vi "FlattenFRF.vi"(9 "CrsrList":T1, 11 "Data in":cluster{"t0":dbl, "dt":dbl, "Y":cdb[]}) -> (1 "Data out":cluster{"t0":dbl, "dt":dbl, "Y":cdb[]})   [LabVIEW 2022 SP3]
uses:
  <vilib>/Utility/miscctls.llb/LVCursorListTypeDef.ctl
panel:
  out "FRF":cluster{"t0":dbl, "dt":dbl, "Y":dbl[]}[](graph)
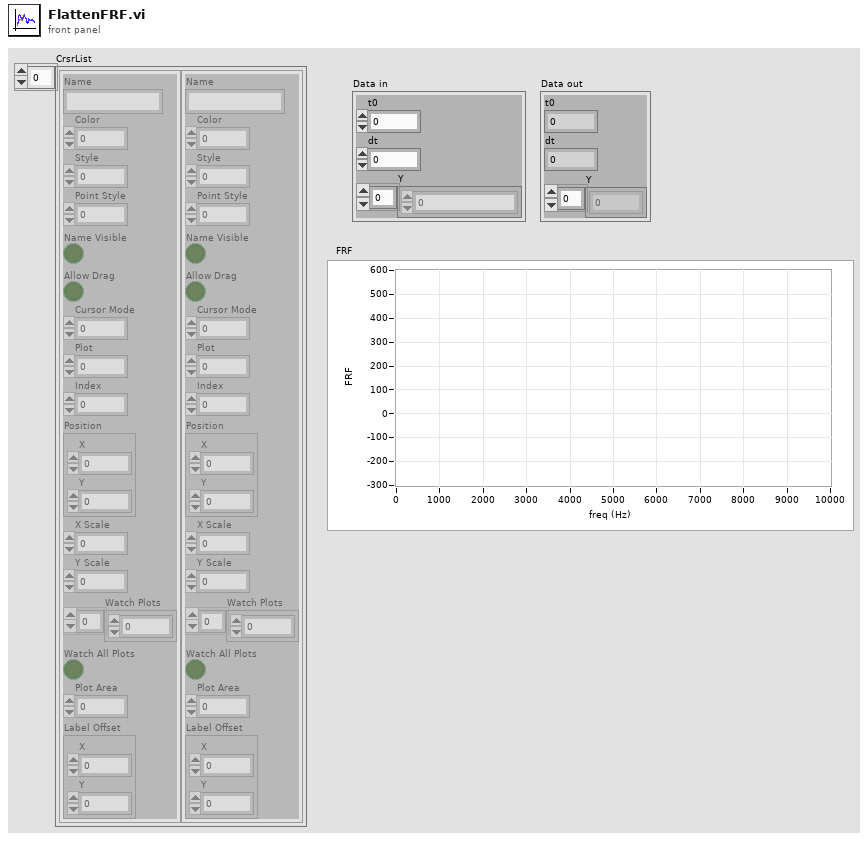
[diagram p1: front panel]
types:
  T1 = typedef "LVCursorListTypeDef.ctl" = cluster{"Name":string, "Color":u32, "Style":u8, "Point Style":u8, "Name Visible":bool, "Allow Drag":bool, "Cursor Mode":u32, "Plot":i32, "Index":i32, "Position":cluster{"X":dbl, "Y":dbl}, "X Scale":u32, "Y Scale":u32, "Watch Plots":i32[], "Watch All Plots":bool, "Plot Area":i32, "Label Offset":cluster{"X":dbl, "Y":dbl}}[]
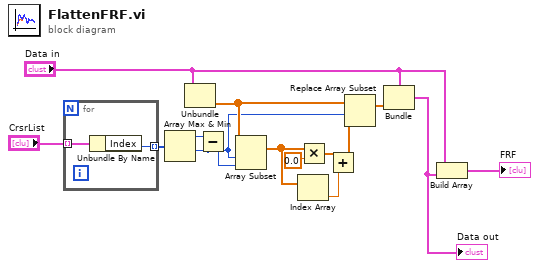
[diagram p0: block diagram]
diagram:
  n1 = for {
    tunnel: "CrsrList" -> [w17] mode=indexing
    tunnel: [w16] -> w12 mode=indexing
    n2 = Unbundle By Name(w17) -> ("Index"=w16:i32)
  }
  n3 = Array Max & Min(array=w12) -> (max value=w9:i32, min value=w10:i32)  [unwired: 2 out]
  n4 = Unbundle("Data in") -> ("Y"=w11:cdb[])  [unwired: 2 out]
  n5 = Subtract(x=w9, y=w10) -> (x-y=w8:i32)
  n6 = Array Subset(array=w11, index=w10, length=w8) -> (w6:cdb[])
  n7 = Index Array(array=w6) -> (element=w5:cdb)  [unwired: 1 in]
  n8 = Multiply(x=w6, y=0.0) -> (x*y=w7:cdb[])
  n9 = Add(x=w7, y=w5) -> (x+y=w4:cdb[])
  n10 = Replace Array Subset(array=w11, new element=w4, index=w10) -> (w13:cdb[])
  n11 = Bundle(cluster="Data in", "Y"=w13) -> (w2:cluster{"t0":dbl, "dt":dbl, "Y":cdb[]})  [unwired: 2 in]
  "Data out" <- w2
  n12 = Build Array("Data in", w2) -> (→"FRF":cluster{"t0":dbl, "dt":dbl, "Y":cdb[]}[])
